vi "Display Lab Panel V6.vi"() -> ()   [LabVIEW 2013]
uses:
  Global display 1.vi
  Global display 2.vi
  Global display 3.vi
panel:
  in  "Tab Control 2":T1(tab)
  out "SIG LAB05-2":T2 {"PF" format="%.2f"; "AMPS" format="%.1f"}
  out "SIG LAB05-1":T2 {"PF" format="%.2f"; "AMPS" format="%.1f"}
  out "SIG LAB04-2":T2 {"PF" format="%.2f"; "AMPS" format="%.1f"}
  out "SIG LAB04-1":T2 {"PF" format="%.2f"; "AMPS" format="%.1f"}
  out "SIG LAB03-2":T2 {"PF" format="%.2f"; "AMPS" format="%.1f"}
  out "SIG LAB03-1":T2 {"PF" format="%.2f"; "AMPS" format="%.1f"}
  out "SIG LAB02-2":T2 {"PF" format="%.2f"; "AMPS" format="%.1f"}
  in  "RUN LAB01-1":bool
  in  "O/I  LAB05-1":bool
  in  "O/I  LAB05-2":bool
  in  "O/I  LAB04-1":bool
  in  "O/I  LAB04-2":bool
  in  "O/I  LAB02-1":bool
  in  "O/I  LAB02-2":bool
  in  "O/I  LAB01-2":bool
  in  "O/I  LAB01-1":bool
  in  "O/I  LAB03-1":bool
  in  "RUN LAB05-2":bool
  in  "RUN LAB05-1":bool
  in  "RUN LAB04-2":bool
  in  "RUN LAB04-1":bool
  in  "RUN LAB03-2":bool
  in  "RUN LAB03-1":bool
  in  "RUN LAB02-2":bool
  in  "RUN LAB02-1":bool
  in  "RUN LAB01-2":bool
  in  "SELECT LAB05-2":T3(radio)
  in  "SELECT LAB05-1":T3(radio)
  in  "SELECT LAB04-2":T3(radio)
  in  "SELECT LAB04-1":T3(radio)
  in  "SELECT LAB03-2":T3(radio)
  in  "SELECT LAB03-1":T3(radio)
  in  "SELECT LAB02-2":T3(radio)
  in  "SELECT LAB02-1":T3(radio)
  in  "SELECT LAB01-2":T3(radio)
  in  "SELECT LAB01-1":T3(radio)
  in  "O/I  LAB03-2":bool
  out "SIG LAB01-1":T2 {"PF" format="%.2f"; "AMPS" format="%.1f"}
  out "SIG LAB01-2":T2 {"PF" format="%.2f"; "AMPS" format="%.1f"}
  out "SIG LAB02-1":T2 {"PF" format="%.2f"; "AMPS" format="%.1f"}
  out "DISP LAB05-2":T4 {"MINS" format="%.2g"}
  out "DISP LAB05-1":T4 {"MINS" format="%.2g"}
  out "DISP LAB04-2":T4 {"MINS" format="%.2g"}
  out "DISP LAB04-1":T4 {"MINS" format="%.2g"}
  out "DISP LAB03-2":T4 {"MINS" format="%.2g"}
  out "DISP LAB03-1":T4 {"MINS" format="%.2g"}
  in  "SET LAB05-2":T5={"NAME"="", "DESCRIPTION"="", "CYCLES"=5.0, "T-RISE mins"=0.0, "T-RISE deg C"=0.0} {"CYCLES" min=5.0 step=1.0}
  in  "SET LAB05-1":T5={"NAME"="", "DESCRIPTION"="", "CYCLES"=5.0, "T-RISE mins"=0.0, "T-RISE deg C"=0.0} {"CYCLES" min=5.0 step=1.0}
  in  "SET LAB04-2":T5={"NAME"="", "DESCRIPTION"="", "CYCLES"=5.0, "T-RISE mins"=0.0, "T-RISE deg C"=0.0} {"CYCLES" min=5.0 step=1.0}
  in  "SET LAB04-1":T5={"NAME"="", "DESCRIPTION"="", "CYCLES"=5.0, "T-RISE mins"=0.0, "T-RISE deg C"=0.0} {"CYCLES" min=5.0 step=1.0}
  in  "SET LAB03-2":T5={"NAME"="", "DESCRIPTION"="", "CYCLES"=5.0, "T-RISE mins"=0.0, "T-RISE deg C"=0.0} {"CYCLES" min=5.0 step=1.0}
  in  "SET LAB03-1":T5={"NAME"="", "DESCRIPTION"="", "CYCLES"=5.0, "T-RISE mins"=0.0, "T-RISE deg C"=0.0} {"CYCLES" min=5.0 step=1.0}
  out "DISP LAB02-2":T4 {"MINS" format="%.2g"}
  out "DISP LAB02-1":T4 {"MINS" format="%.2g"}
  in  "SET LAB02-2":T5={"NAME"="", "DESCRIPTION"="", "CYCLES"=5.0, "T-RISE mins"=0.0, "T-RISE deg C"=0.0} {"CYCLES" min=5.0 step=1.0}
  in  "SET LAB02-1":T5={"NAME"="", "DESCRIPTION"="", "CYCLES"=5.0, "T-RISE mins"=0.0, "T-RISE deg C"=0.0} {"CYCLES" min=5.0 step=1.0}
  out "RESULT LAB05-2":bool
  out "RESULT LAB05-1":bool
  out "RESULT LAB04-2":bool
  out "RESULT LAB04-1":bool
  out "RESULT LAB03-2":bool
  out "RESULT LAB03-1":bool
  out "RESULT LAB02-2":bool
  out "RESULT LAB02-1":bool
  out "RESULT LAB01-2":bool
  out "RESULT LAB01-1":bool
  in  "SET LAB01-1":T5={"NAME"="", "DESCRIPTION"="", "CYCLES"=5.0, "T-RISE mins"=0.0, "T-RISE deg C"=0.0} {"CYCLES" min=5.0 step=1.0}
  in  "SET LAB01-2":T5={"NAME"="", "DESCRIPTION"="", "CYCLES"=5.0, "T-RISE mins"=0.0, "T-RISE deg C"=0.0} {"CYCLES" min=5.0 step=1.0}
  out "DISP LAB01-1":T4 {"MINS" format="%.2g"}
  out "DISP LAB01-2":T4 {"MINS" format="%.2f"}
  in  "Save Log Files\nTo Disk For\nViewing":bool
  out "LOG LAB05-2":string
  out "LOG LAB04-2":string
  out "LOG LAB03-2":string
  out "LOG LAB02-2":string
  out "LOG LAB01-2":string
  out "LOG LAB05-1":string
  out "LOG LAB04-1":string
  out "LOG LAB03-1":string
  out "LOG LAB02-1":string
  out "LOG LAB01-1":string
  out "LAB01 TEMP":dynamicdata(graph)
  out "LAB01 VOLTS":dynamicdata(graph)
  out "LAB01 AMPS":dynamicdata(graph)
  out "LAB02 TEMP":dynamicdata(graph)
  out "LAB02 VOLTS":dynamicdata(graph)
  out "LAB02 AMPS":dynamicdata(graph)
  out "LAB03 TEMP":dynamicdata(graph)
  out "LAB03 VOLTS":dynamicdata(graph)
  out "LAB03 AMPS":dynamicdata(graph)
  out "LAB04 TEMP":dynamicdata(graph)
  out "LAB04 VOLTS":dynamicdata(graph)
  out "LAB04 AMPS":dynamicdata(graph)
  out "LAB05 TEMP":dynamicdata(graph)
  out "LAB05 VOLTS":dynamicdata(graph)
  out "LAB05 AMPS":dynamicdata(graph)
  in  "Stop Button":bool
  out "log file dir":string
  out "log5-2":dbl
  out "log4-2":dbl
  out "log3-2":dbl
  out "log2-2":dbl
  out "log1-2":dbl
  out "log5-1":dbl
  out "log4-1":dbl
  out "log3-1":dbl
  out "log2-1":dbl
  out "log1-1":dbl
  out "graph update":bool
  out "LF5-2":bool
  out "LF5-1":bool
  out "LF3-2":bool
  out "LF3-1":bool
  out "LF4-2":bool
  out "LF4-1":bool
  out "LF2-2":bool
  out "LF2-1":bool
  out "LF1-2":bool
  out "LF1-1":bool
  out "error out":errorcluster
  # "LAB01"
  # "LAB02"
  # "LAB05"
  # "LAB03"
  # "LAB04"
  # "LAB01"
  # "LAB02"
  # "LAB03"
  # "LAB04"
  # "LAB05"
  # "PANEL ID / DATE / TIME / DESCRIPTION / CYCLES / TEST TIME / STATUS"
  # "PANEL ID / DATE / TIME / DESCRIPTION / CYCLES / TEST TIME / STATUS"
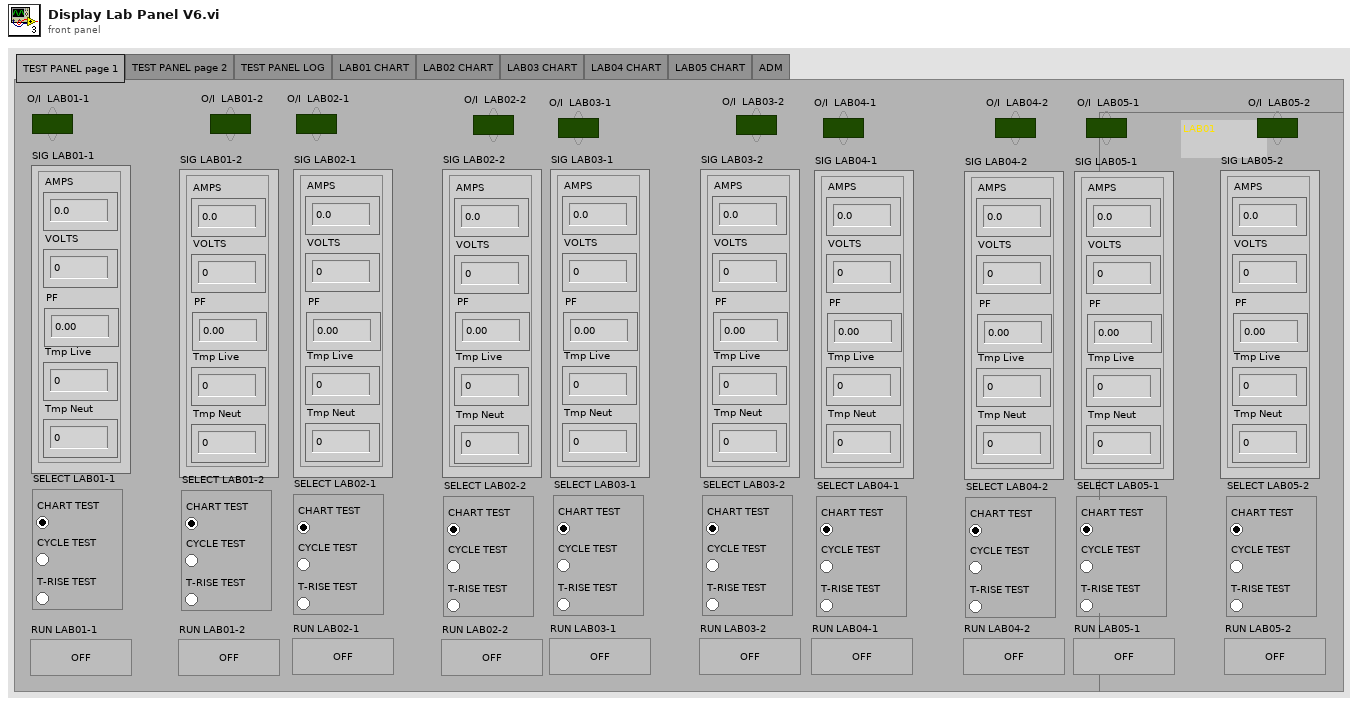
[diagram p1: front panel]
types:
  T1 = enum32{"TEST PANEL page 1", "TEST PANEL page 2", "TEST PANEL LOG", "LAB01 CHART", "LAB02 CHART", "LAB03 CHART", "LAB04 CHART", "LAB05 CHART", "ADM"}
  T2 = cluster{"AMPS":dbl, "VOLTS":dbl, "PF":dbl, "Tmp Live":dbl, "Tmp Neut":dbl}
  T3 = enum32{"CHART TEST", "CYCLE TEST", "T-RISE TEST"}
  T4 = cluster{"CYCLE":dbl, "MINS":dbl, "STATUS":string}
  T5 = cluster{"NAME":string, "DESCRIPTION":string, "CYCLES":dbl, "T-RISE mins":dbl, "T-RISE deg C":dbl}
  T6 = enum8{"Enabled", "Disabled", "Disabled and Grayed Out"}
  T7 = cluster{string, "date string":string, "time string":string, "DESCRIPTION":string, string, string, "STATUS":string}
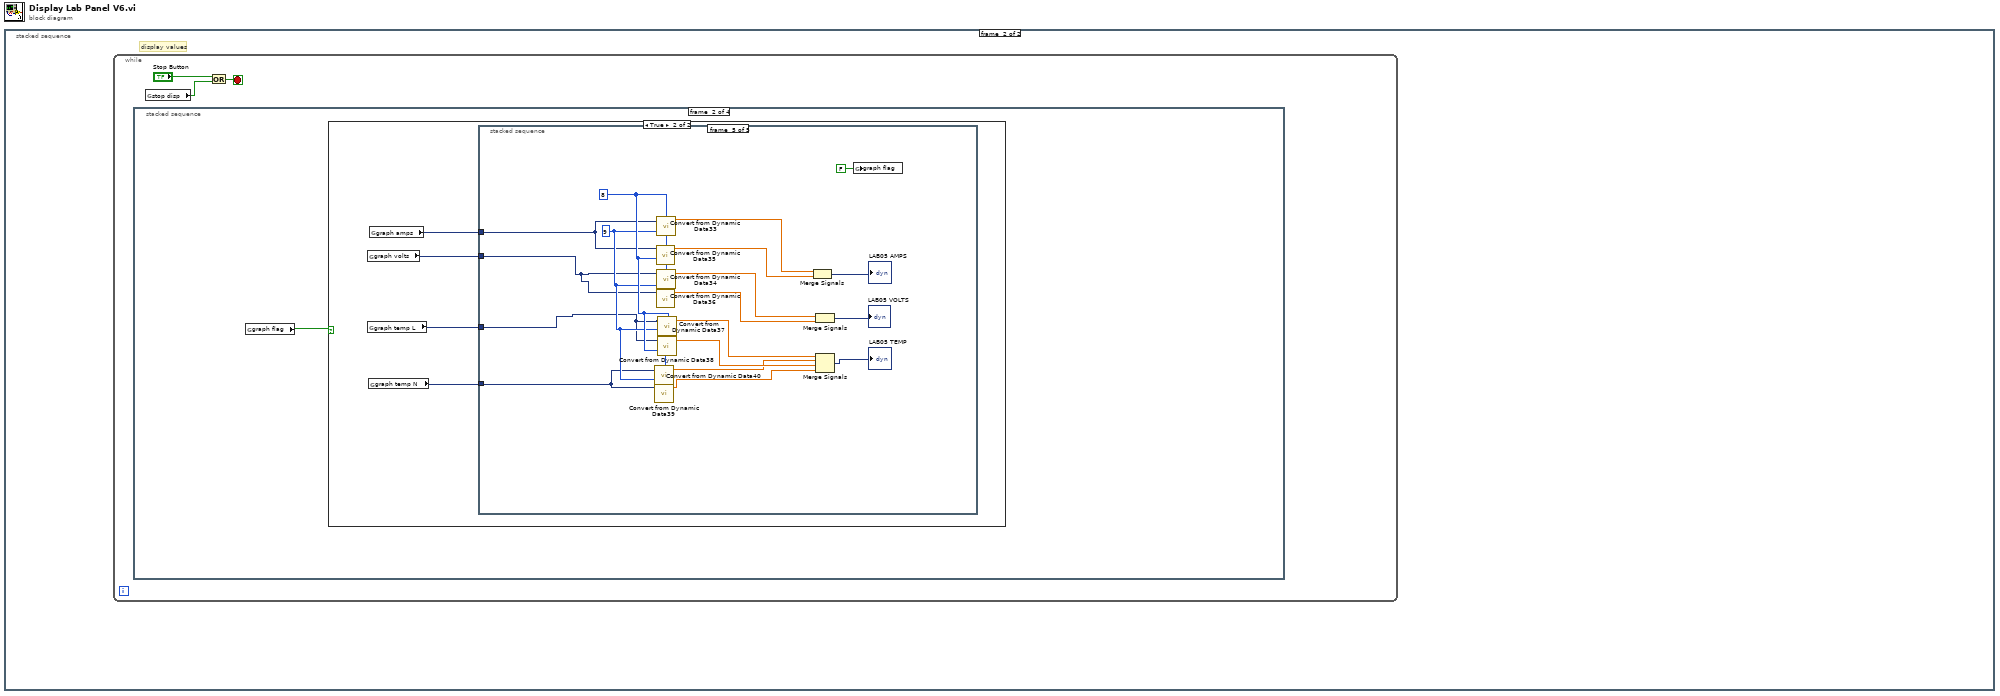
[diagram p0: block diagram]
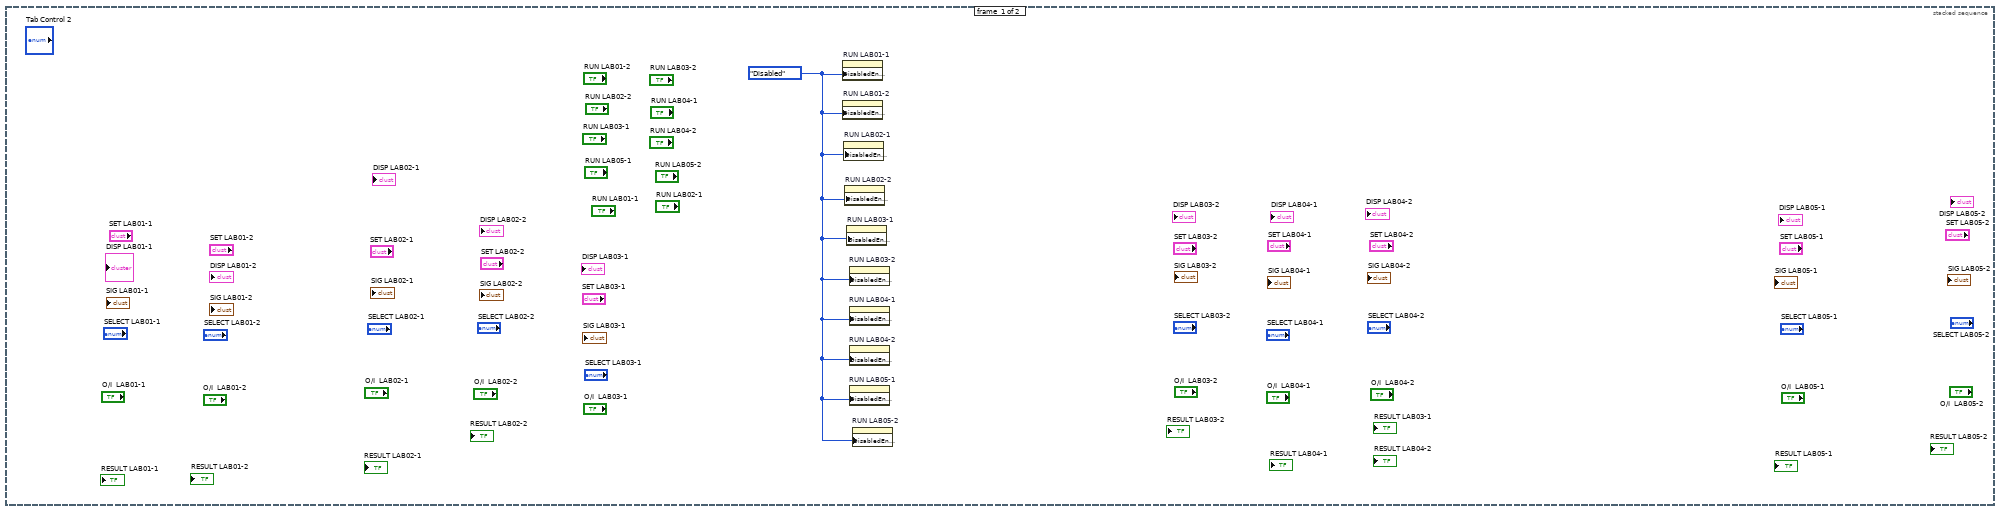
[diagram p2: hidden frame]
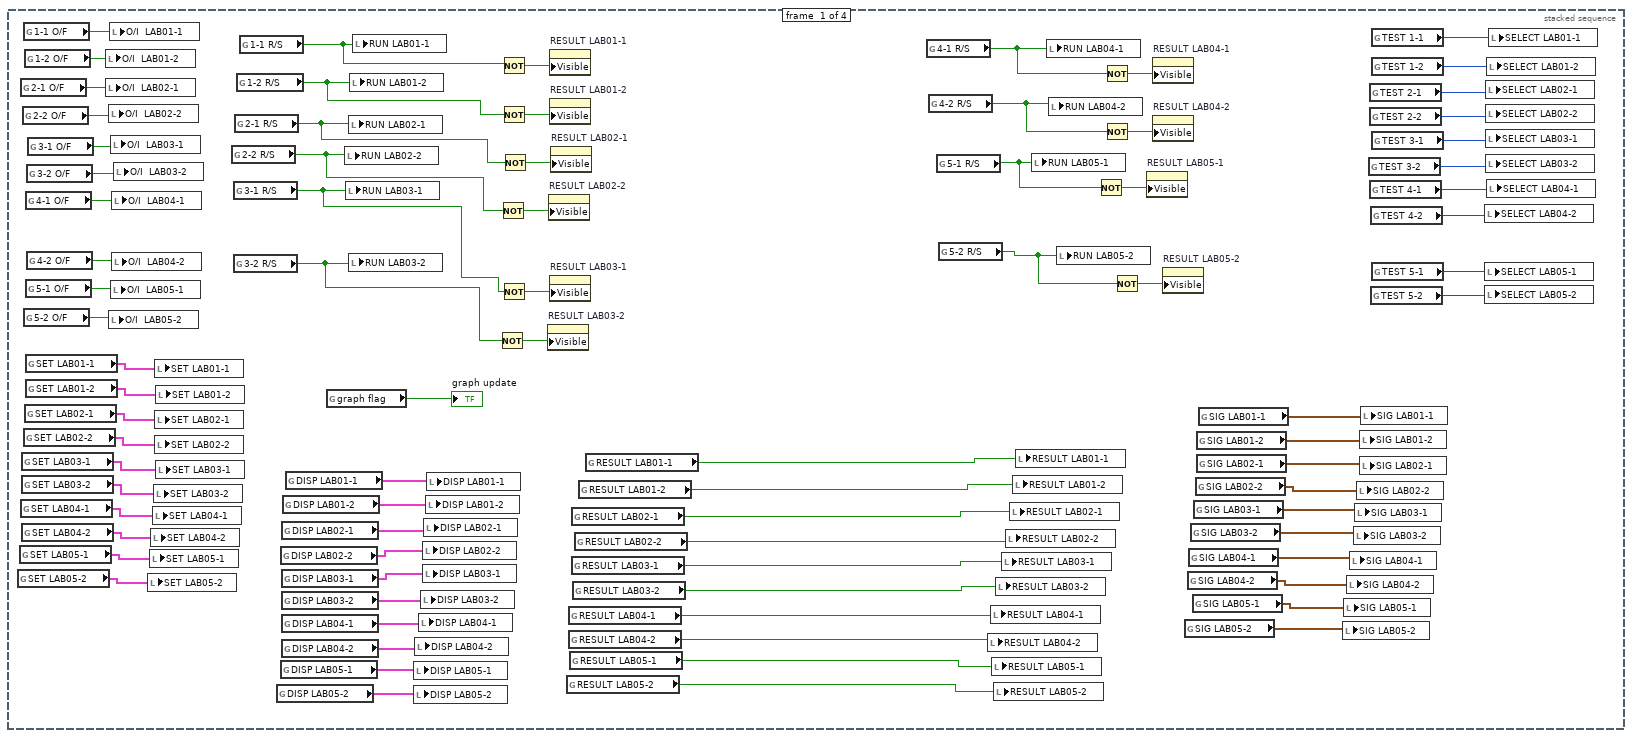
[diagram p3: hidden frame]
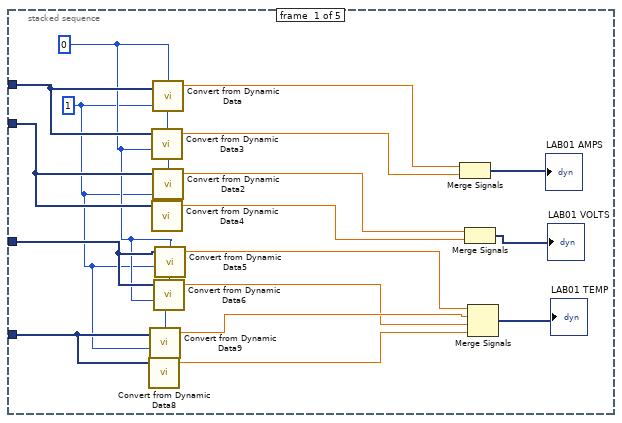
[diagram p5: hidden frame]
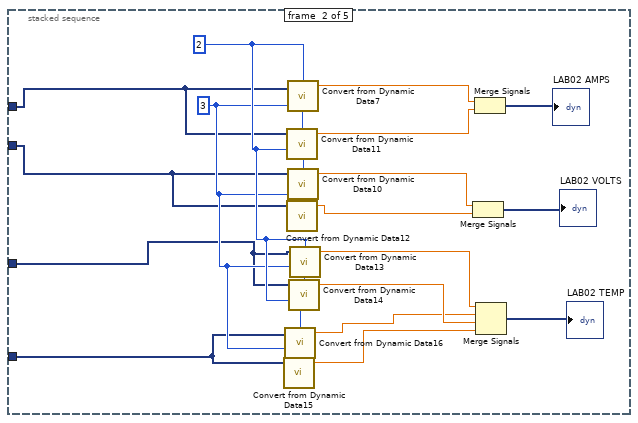
[diagram p6: hidden frame]
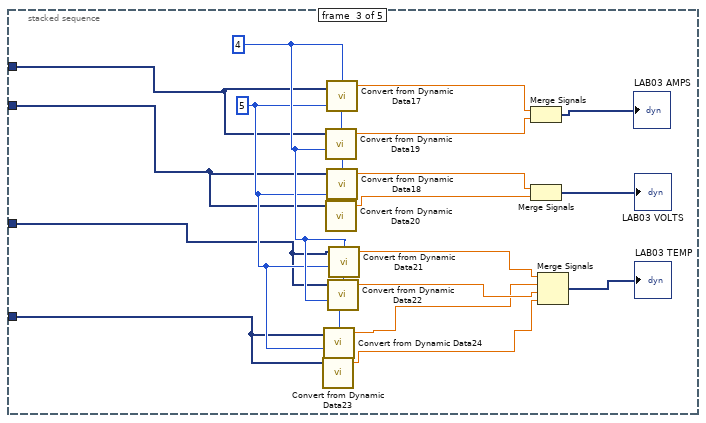
[diagram p7: hidden frame]
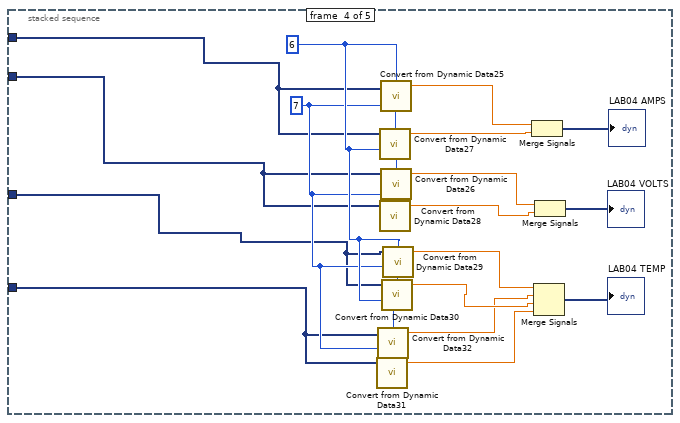
[diagram p8: hidden frame]
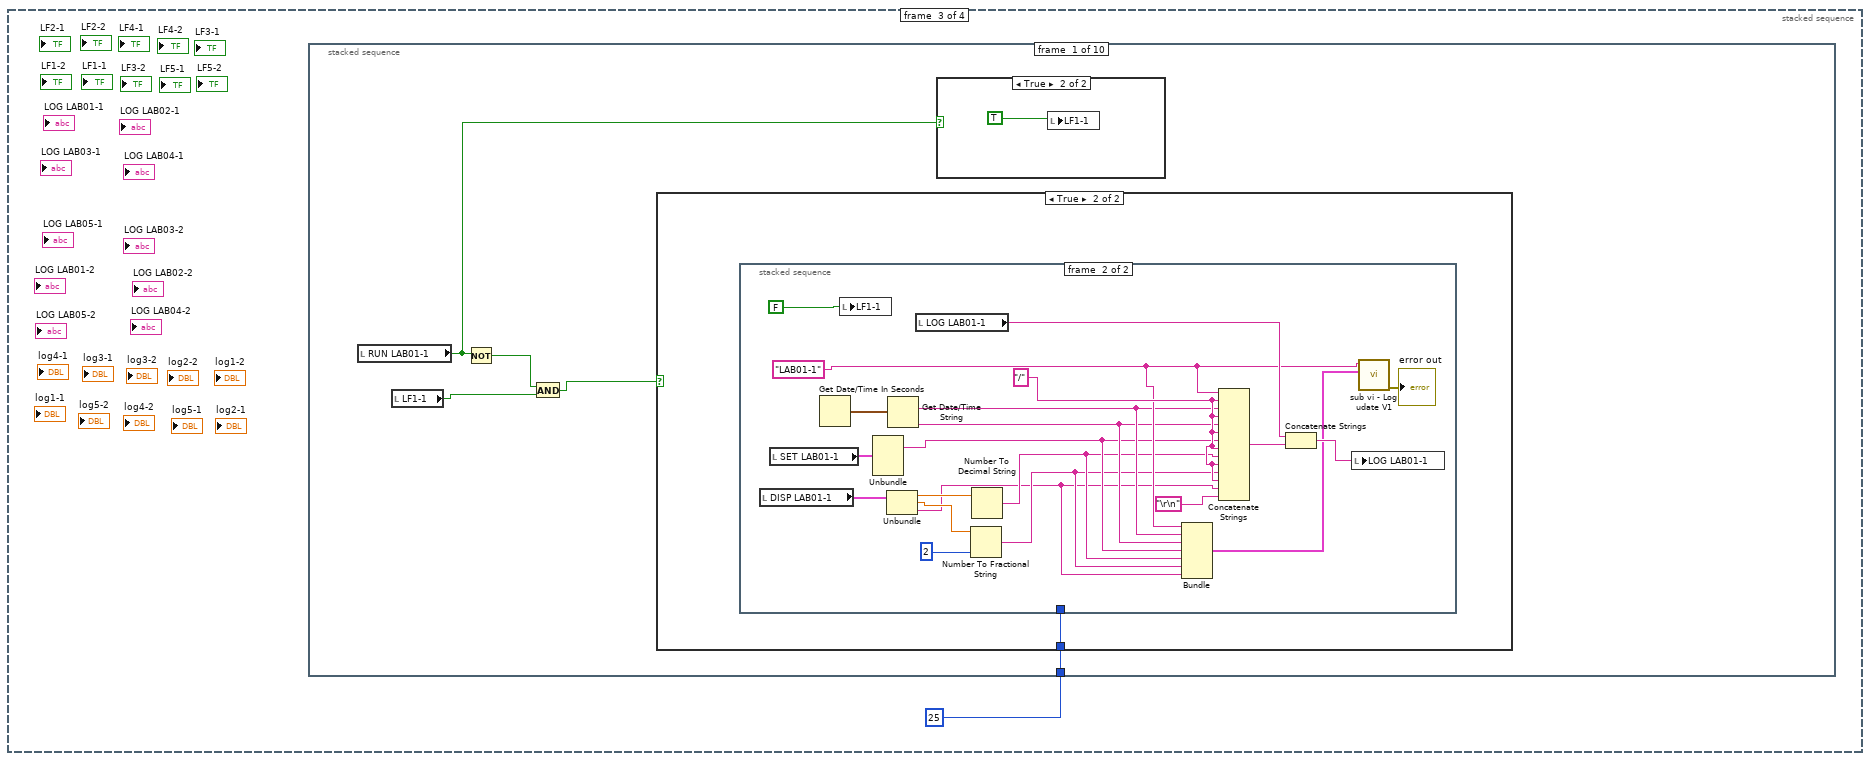
[diagram p9: hidden frame]
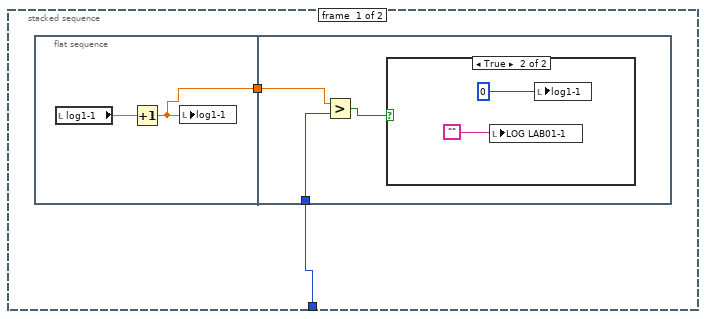
[diagram p11: hidden frame]
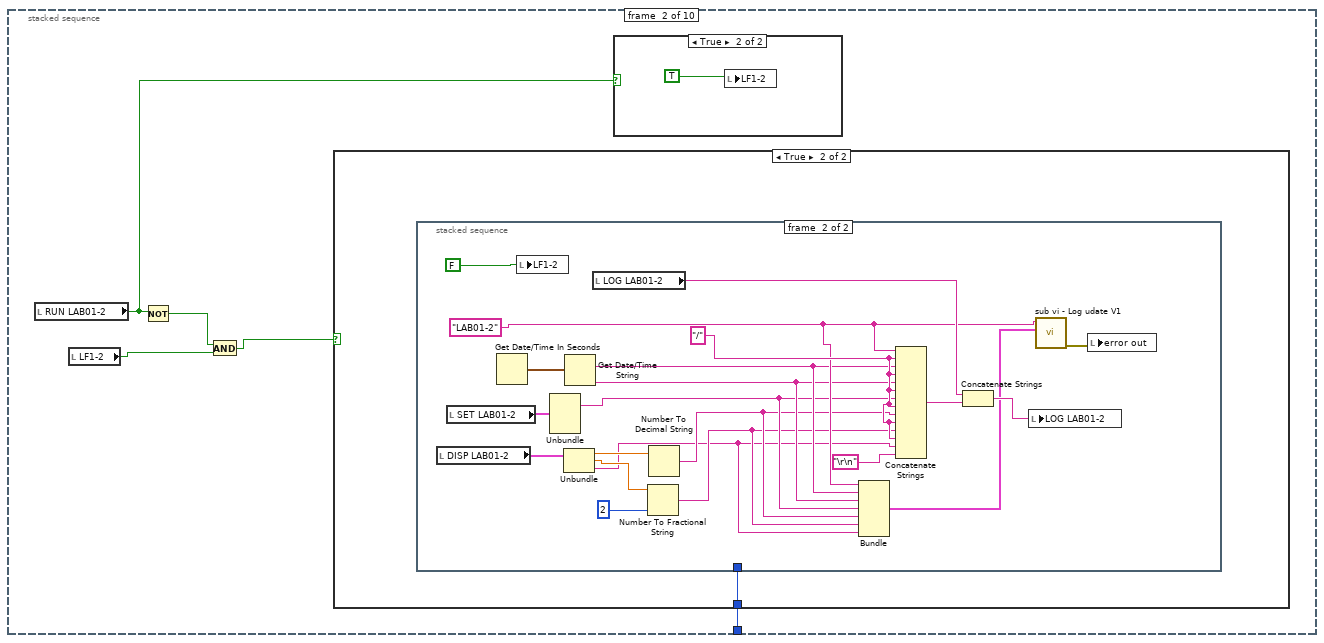
[diagram p14: hidden frame]
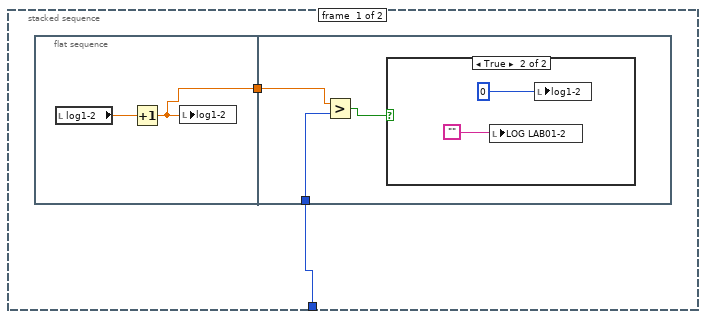
[diagram p16: hidden frame]
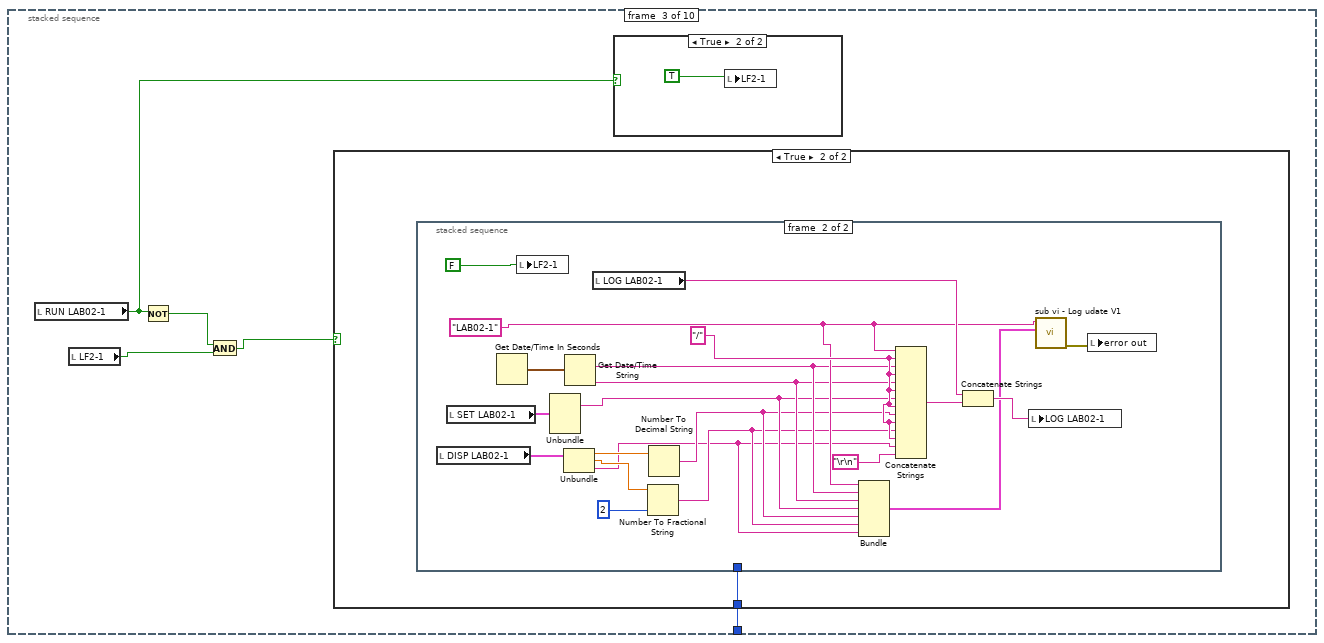
[diagram p19: hidden frame]
diagram:
  n1 = stacked-sequence {
    frame #0 {
      w1 = T6."Disabled" ("Disabled")
      n2 = property on="RUN LAB01-1" class="Bool (strict)"("DisabledEnum"=w1) -> ()  [unwired: 2 in, 2 out]
      n3 = property on="RUN LAB01-2" class="Bool (strict)"("DisabledEnum"=w1) -> ()  [unwired: 2 in, 2 out]
      n4 = property on="RUN LAB02-1" class="Bool (strict)"("DisabledEnum"=w1) -> ()  [unwired: 2 in, 2 out]
      n5 = property on="RUN LAB02-2" class="Bool (strict)"("DisabledEnum"=w1) -> ()  [unwired: 2 in, 2 out]
      n6 = property on="RUN LAB03-1" class="Bool (strict)"("DisabledEnum"=w1) -> ()  [unwired: 2 in, 2 out]
      n7 = property on="RUN LAB03-2" class="Bool (strict)"("DisabledEnum"=w1) -> ()  [unwired: 2 in, 2 out]
      n8 = property on="RUN LAB04-1" class="Bool (strict)"("DisabledEnum"=w1) -> ()  [unwired: 2 in, 2 out]
      n9 = property on="RUN LAB04-2" class="Bool (strict)"("DisabledEnum"=w1) -> ()  [unwired: 2 in, 2 out]
      n10 = property on="RUN LAB05-1" class="Bool (strict)"("DisabledEnum"=w1) -> ()  [unwired: 2 in, 2 out]
      n11 = property on="RUN LAB05-2" class="Bool (strict)"("DisabledEnum"=w1) -> ()  [unwired: 2 in, 2 out]
    }
    frame #1 {
      # "display values"
      n12 = while {
        stop <- w4 stop-if-true
        n13 = stacked-sequence {
          frame #0 {
            n14 = global read "Global display 2.vi" "SET LAB05-2"() -> (w46:T5)
            n15 = global read "Global display 2.vi" "SET LAB05-1"() -> (w47:T5)
            n16 = global read "Global display 1.vi" "2-1 O/F"() -> (w83:bool)
            n17 = global read "Global display 2.vi" "SET LAB04-1"() -> (w49:T5)
            n18 = global read "Global display 2.vi" "SET LAB03-1"() -> (w51:T5)
            n19 = global read "Global display 2.vi" "SET LAB03-2"() -> (w50:T5)
            n20 = global read "Global display 2.vi" "SET LAB04-2"() -> (w48:T5)
            n21 = global read "Global display 1.vi" "2-2 O/F"() -> (w82:bool)
            n22 = global read "Global display 1.vi" "1-1 O/F"() -> (w85:bool)
            n23 = global read "Global display 1.vi" "5-2 O/F"() -> (w76:bool)
            n24 = global read "Global display 2.vi" "SET LAB02-2"() -> (w52:T5)
            n25 = global read "Global display 1.vi" "1-2 O/F"() -> (w84:bool)
            n26 = global read "Global display 2.vi" "SET LAB02-1"() -> (w53:T5)
            n27 = global read "Global display 1.vi" "4-1 O/F"() -> (w79:bool)
            n28 = global read "Global display 1.vi" "5-1 O/F"() -> (w77:bool)
            n29 = global read "Global display 2.vi" "SET LAB01-1"() -> (w55:T5)
            n30 = global read "Global display 2.vi" "SET LAB01-2"() -> (w54:T5)
            n31 = global read "Global display 1.vi" "3-2 O/F"() -> (w80:bool)
            n32 = global read "Global display 1.vi" "4-2 O/F"() -> (w78:bool)
            n33 = global read "Global display 1.vi" "3-1 O/F"() -> (w81:bool)
            n34 = local write "O/I  LAB01-2"(w84) -> ()
            n35 = local write "O/I  LAB02-1"(w83) -> ()
            n36 = local write "O/I  LAB02-2"(w82) -> ()
            n37 = local write "O/I  LAB05-2"(w76) -> ()
            n38 = local write "O/I  LAB01-1"(w85) -> ()
            n39 = local write "O/I  LAB03-1"(w81) -> ()
            n40 = local write "O/I  LAB05-1"(w77) -> ()
            n41 = local write "O/I  LAB04-1"(w79) -> ()
            n42 = local write "O/I  LAB04-2"(w78) -> ()
            n43 = local write "O/I  LAB03-2"(w80) -> ()
            n44 = local write "SET LAB05-2"(w46) -> ()
            n45 = local write "SET LAB05-1"(w47) -> ()
            n46 = local write "SET LAB04-2"(w48) -> ()
            n47 = local write "SET LAB04-1"(w49) -> ()
            n48 = local write "SET LAB03-2"(w50) -> ()
            n49 = local write "SET LAB01-1"(w55) -> ()
            n50 = local write "SET LAB02-1"(w53) -> ()
            n51 = local write "SET LAB02-2"(w52) -> ()
            n52 = local write "SET LAB01-2"(w54) -> ()
            n53 = local write "SET LAB03-1"(w51) -> ()
            n54 = global read "Global display 1.vi" "2-2 R/S"() -> (w16:bool)
            n55 = global read "Global display 1.vi" "3-1 R/S"() -> (w15:bool)
            n56 = global read "Global display 1.vi" "3-2 R/S"() -> (w14:bool)
            n57 = global read "Global display 1.vi" "2-1 R/S"() -> (w17:bool)
            n58 = global read "Global display 1.vi" "1-2 R/S"() -> (w18:bool)
            n59 = global read "Global display 1.vi" "1-1 R/S"() -> (w24:bool)
            n60 = global read "Global display 2.vi" "DISP LAB05-2"() -> (w36:T4)
            n61 = global read "Global display 2.vi" "DISP LAB02-2"() -> (w42:T4)
            n62 = global read "Global display 2.vi" "DISP LAB05-1"() -> (w37:T4)
            n63 = global read "Global display 2.vi" "DISP LAB02-1"() -> (w43:T4)
            n64 = global read "Global display 2.vi" "DISP LAB03-1"() -> (w41:T4)
            n65 = global read "Global display 2.vi" "DISP LAB03-2"() -> (w40:T4)
            n66 = global read "Global display 2.vi" "DISP LAB04-1"() -> (w39:T4)
            n67 = global read "Global display 2.vi" "DISP LAB04-2"() -> (w38:T4)
            n68 = global read "Global display 2.vi" "DISP LAB01-2"() -> (w44:T4)
            n69 = global read "Global display 2.vi" "DISP LAB01-1"() -> (w45:T4)
            n70 = global read "Global display 3.vi" "graph flag"() -> (→"graph update":bool)
            n71 = local write "RUN LAB02-2"(w16) -> ()
            n72 = local write "RUN LAB03-1"(w15) -> ()
            n73 = local write "RUN LAB02-1"(w17) -> ()
            n74 = local write "RUN LAB03-2"(w14) -> ()
            n75 = local write "RUN LAB01-2"(w18) -> ()
            n76 = local write "RUN LAB01-1"(w24) -> ()
            n77 = local write "DISP LAB05-1"(w37) -> ()
            n78 = local write "DISP LAB05-2"(w36) -> ()
            n79 = local write "DISP LAB04-2"(w38) -> ()
            n80 = local write "DISP LAB04-1"(w39) -> ()
            n81 = local write "DISP LAB03-2"(w40) -> ()
            n82 = local write "DISP LAB02-2"(w42) -> ()
            n83 = local write "DISP LAB03-1"(w41) -> ()
            n84 = local write "DISP LAB02-1"(w43) -> ()
            n85 = local write "DISP LAB01-2"(w44) -> ()
            n86 = local write "DISP LAB01-1"(w45) -> ()
            n87 = Not(x=w14) -> (.not. x?=w19:bool)
            n88 = Not(x=w16) -> (.not. x?=w21:bool)
            n89 = Not(x=w24) -> (.not. x?=w25:bool)
            n90 = Not(x=w18) -> (.not. x?=w23:bool)
            n91 = Not(x=w15) -> (.not. x?=w20:bool)
            n92 = Not(x=w17) -> (.not. x?=w22:bool)
            n93 = property on="RESULT LAB03-2" class="Bool (strict)"("Visible"=w19) -> ()  [unwired: 2 in, 2 out]
            n94 = property on="RESULT LAB02-2" class="Bool (strict)"("Visible"=w21) -> ()  [unwired: 2 in, 2 out]
            n95 = property on="RESULT LAB01-1" class="Bool (strict)"("Visible"=w25) -> ()  [unwired: 2 in, 2 out]
            n96 = property on="RESULT LAB01-2" class="Bool (strict)"("Visible"=w23) -> ()  [unwired: 2 in, 2 out]
            n97 = property on="RESULT LAB03-1" class="Bool (strict)"("Visible"=w20) -> ()  [unwired: 2 in, 2 out]
            n98 = property on="RESULT LAB02-1" class="Bool (strict)"("Visible"=w22) -> ()  [unwired: 2 in, 2 out]
            n99 = global read "Global display 2.vi" "RESULT LAB05-2"() -> (w26:bool)
            n100 = global read "Global display 2.vi" "RESULT LAB04-1"() -> (w29:bool)
            n101 = global read "Global display 2.vi" "RESULT LAB04-2"() -> (w28:bool)
            n102 = global read "Global display 2.vi" "RESULT LAB05-1"() -> (w27:bool)
            n103 = global read "Global display 2.vi" "RESULT LAB02-1"() -> (w33:bool)
            n104 = global read "Global display 2.vi" "RESULT LAB03-1"() -> (w31:bool)
            n105 = global read "Global display 2.vi" "RESULT LAB03-2"() -> (w30:bool)
            n106 = global read "Global display 2.vi" "RESULT LAB02-2"() -> (w32:bool)
            n107 = global read "Global display 2.vi" "RESULT LAB01-2"() -> (w34:bool)
            n108 = global read "Global display 2.vi" "RESULT LAB01-1"() -> (w35:bool)
            n109 = global read "Global display 1.vi" "4-1 R/S"() -> (w12:bool)
            n110 = global read "Global display 1.vi" "4-2 R/S"() -> (w10:bool)
            n111 = global read "Global display 1.vi" "5-1 R/S"() -> (w8:bool)
            n112 = global read "Global display 1.vi" "5-2 R/S"() -> (w6:bool)
            n113 = local write "RESULT LAB04-2"(w28) -> ()
            n114 = local write "RESULT LAB04-1"(w29) -> ()
            n115 = local write "RESULT LAB05-1"(w27) -> ()
            n116 = local write "RESULT LAB05-2"(w26) -> ()
            n117 = local write "RESULT LAB03-2"(w30) -> ()
            n118 = local write "RESULT LAB03-1"(w31) -> ()
            n119 = local write "RESULT LAB02-2"(w32) -> ()
            n120 = local write "RESULT LAB02-1"(w33) -> ()
            n121 = local write "RESULT LAB01-2"(w34) -> ()
            n122 = local write "RESULT LAB01-1"(w35) -> ()
            n123 = local write "RUN LAB05-1"(w8) -> ()
            n124 = local write "RUN LAB04-1"(w12) -> ()
            n125 = local write "RUN LAB04-2"(w10) -> ()
            n126 = local write "RUN LAB05-2"(w6) -> ()
            n127 = Not(x=w8) -> (.not. x?=w9:bool)
            n128 = Not(x=w12) -> (.not. x?=w13:bool)
            n129 = Not(x=w10) -> (.not. x?=w11:bool)
            n130 = Not(x=w6) -> (.not. x?=w7:bool)
            n131 = property on="RESULT LAB05-1" class="Bool (strict)"("Visible"=w9) -> ()  [unwired: 2 in, 2 out]
            n132 = property on="RESULT LAB04-1" class="Bool (strict)"("Visible"=w13) -> ()  [unwired: 2 in, 2 out]
            n133 = property on="RESULT LAB04-2" class="Bool (strict)"("Visible"=w11) -> ()  [unwired: 2 in, 2 out]
            n134 = property on="RESULT LAB05-2" class="Bool (strict)"("Visible"=w7) -> ()  [unwired: 2 in, 2 out]
            n135 = global read "Global display 1.vi" "SIG LAB05-2"() -> (w56:T2)
            n136 = global read "Global display 1.vi" "SIG LAB04-2"() -> (w58:T2)
            n137 = global read "Global display 1.vi" "SIG LAB04-1"() -> (w59:T2)
            n138 = global read "Global display 1.vi" "SIG LAB03-2"() -> (w60:T2)
            n139 = global read "Global display 1.vi" "SIG LAB05-1"() -> (w57:T2)
            n140 = global read "Global display 1.vi" "SIG LAB03-1"() -> (w61:T2)
            n141 = global read "Global display 1.vi" "SIG LAB02-2"() -> (w62:T2)
            n142 = global read "Global display 1.vi" "SIG LAB01-2"() -> (w64:T2)
            n143 = global read "Global display 1.vi" "SIG LAB02-1"() -> (w63:T2)
            n144 = global read "Global display 1.vi" "SIG LAB01-1"() -> (w65:T2)
            n145 = local write "SIG LAB05-2"(w56) -> ()
            n146 = local write "SIG LAB05-1"(w57) -> ()
            n147 = local write "SIG LAB04-2"(w58) -> ()
            n148 = local write "SIG LAB04-1"(w59) -> ()
            n149 = local write "SIG LAB03-2"(w60) -> ()
            n150 = local write "SIG LAB03-1"(w61) -> ()
            n151 = local write "SIG LAB02-2"(w62) -> ()
            n152 = local write "SIG LAB01-2"(w64) -> ()
            n153 = local write "SIG LAB02-1"(w63) -> ()
            n154 = local write "SIG LAB01-1"(w65) -> ()
            n155 = global read "Global display 1.vi" "TEST 3-2"() -> (w70:T3)
            n156 = global read "Global display 1.vi" "TEST 2-1"() -> (w73:T3)
            n157 = global read "Global display 1.vi" "TEST 2-2"() -> (w72:T3)
            n158 = global read "Global display 1.vi" "TEST 4-1"() -> (w69:T3)
            n159 = global read "Global display 1.vi" "TEST 4-2"() -> (w68:T3)
            n160 = global read "Global display 1.vi" "TEST 5-2"() -> (w66:T3)
            n161 = global read "Global display 1.vi" "TEST 1-1"() -> (w75:T3)
            n162 = global read "Global display 1.vi" "TEST 1-2"() -> (w74:T3)
            n163 = global read "Global display 1.vi" "TEST 3-1"() -> (w71:T3)
            n164 = global read "Global display 1.vi" "TEST 5-1"() -> (w67:T3)
            n165 = local write "SELECT LAB04-2"(w68) -> ()
            n166 = local write "SELECT LAB05-1"(w67) -> ()
            n167 = local write "SELECT LAB05-2"(w66) -> ()
            n168 = local write "SELECT LAB02-1"(w73) -> ()
            n169 = local write "SELECT LAB02-2"(w72) -> ()
            n170 = local write "SELECT LAB03-1"(w71) -> ()
            n171 = local write "SELECT LAB03-2"(w70) -> ()
            n172 = local write "SELECT LAB01-2"(w74) -> ()
            n173 = local write "SELECT LAB04-1"(w69) -> ()
            n174 = local write "SELECT LAB01-1"(w75) -> ()
          }
          frame #1 {
            n175 = global read "Global display 3.vi" "graph flag"() -> (w86:bool)
            n176 = case shown="True" w86 {
              frame False {
              }
              frame True {
                n177 = global read "Global display 3.vi" "graph volts"() -> (w89:dynamicdata)
                n178 = global read "Global display 3.vi" "graph temp L"() -> (w88:dynamicdata)
                n179 = global read "Global display 3.vi" "graph temp N"() -> (w87:dynamicdata)
                n180 = global read "Global display 3.vi" "graph amps"() -> (w90:dynamicdata)
                n181 = stacked-sequence {
                  tunnel: w90 -> [w104 w119 w136 w153 w170]
                  tunnel: w89 -> [w101 w116 w135 w152 w169]
                  tunnel: w88 -> [w98 w118 w134 w151 w168]
                  tunnel: w87 -> [w97 w117 w133 w150 w167]
                  frame #0 {
                    w91 = 1
                    w96 = 0
                    n182 = call "Convert from Dynamic Data8"("Dynamic Data Type"=w97, "Channel"=w91) -> ("Scalar"=w92:dbl)  [unwired: 2 in]
                    n183 = call "Convert from Dynamic Data9"("Dynamic Data Type"=w97, "Channel"=w96) -> ("Scalar"=w94:dbl)  [unwired: 2 in]
                    n184 = call "Convert from Dynamic Data3"("Dynamic Data Type"=w104, "Channel"=w91) -> ("Scalar"=w102:dbl)  [unwired: 2 in]
                    n185 = call "Convert from Dynamic Data4"("Dynamic Data Type"=w101, "Channel"=w91) -> ("Scalar"=w99:dbl)  [unwired: 2 in]
                    n186 = call "Convert from Dynamic Data"("Dynamic Data Type"=w104, "Channel"=w96) -> ("Scalar"=w103:dbl)  [unwired: 2 in]
                    n187 = call "Convert from Dynamic Data2"("Dynamic Data Type"=w101, "Channel"=w96) -> ("Scalar"=w100:dbl)  [unwired: 2 in]
                    n188 = call "Convert from Dynamic Data6"("Dynamic Data Type"=w98, "Channel"=w91) -> ("Scalar"=w93:dbl)  [unwired: 2 in]
                    n189 = call "Convert from Dynamic Data5"("Dynamic Data Type"=w98, "Channel"=w96) -> ("Scalar"=w95:dbl)  [unwired: 2 in]
                    n190 = Merge Signals(w103, w102) -> (→"LAB01 AMPS":dynamicdata)
                    n191 = Merge Signals(w100, w99) -> (→"LAB01 VOLTS":dynamicdata)
                    n192 = Merge Signals(w95, w94, w93, w92) -> (→"LAB01 TEMP":dynamicdata)
                  }
                  frame #1 {
                    w123 = 3
                    w124 = 2
                    n193 = call "Convert from Dynamic Data15"("Dynamic Data Type"=w117, "Channel"=w123) -> ("Scalar"=w108:dbl)  [unwired: 2 in]
                    n194 = call "Convert from Dynamic Data16"("Dynamic Data Type"=w117, "Channel"=w124) -> ("Scalar"=w109:dbl)  [unwired: 2 in]
                    n195 = call "Convert from Dynamic Data11"("Dynamic Data Type"=w119, "Channel"=w123) -> ("Scalar"=w114:dbl)  [unwired: 2 in]
                    n196 = call "Convert from Dynamic Data12"("Dynamic Data Type"=w116, "Channel"=w123) -> ("Scalar"=w112:dbl)  [unwired: 2 in]
                    n197 = call "Convert from Dynamic Data7"("Dynamic Data Type"=w119, "Channel"=w124) -> ("Scalar"=w115:dbl)  [unwired: 2 in]
                    n198 = call "Convert from Dynamic Data10"("Dynamic Data Type"=w116, "Channel"=w124) -> ("Scalar"=w113:dbl)  [unwired: 2 in]
                    n199 = call "Convert from Dynamic Data14"("Dynamic Data Type"=w118, "Channel"=w123) -> ("Scalar"=w110:dbl)  [unwired: 2 in]
                    n200 = call "Convert from Dynamic Data13"("Dynamic Data Type"=w118, "Channel"=w124) -> ("Scalar"=w111:dbl)  [unwired: 2 in]
                    n201 = Merge Signals(w113, w112) -> (→"LAB02 VOLTS":dynamicdata)
                    n202 = Merge Signals(w115, w114) -> (→"LAB02 AMPS":dynamicdata)
                    n203 = Merge Signals(w111, w109, w110, w108) -> (→"LAB02 TEMP":dynamicdata)
                  }
                  frame #2 {
                    w140 = 5
                    w141 = 4
                    n204 = call "Convert from Dynamic Data23"("Dynamic Data Type"=w133, "Channel"=w140) -> ("Scalar"=w125:dbl)  [unwired: 2 in]
                    n205 = call "Convert from Dynamic Data24"("Dynamic Data Type"=w133, "Channel"=w141) -> ("Scalar"=w126:dbl)  [unwired: 2 in]
                    n206 = call "Convert from Dynamic Data19"("Dynamic Data Type"=w136, "Channel"=w140) -> ("Scalar"=w131:dbl)  [unwired: 2 in]
                    n207 = call "Convert from Dynamic Data20"("Dynamic Data Type"=w135, "Channel"=w140) -> ("Scalar"=w129:dbl)  [unwired: 2 in]
                    n208 = call "Convert from Dynamic Data17"("Dynamic Data Type"=w136, "Channel"=w141) -> ("Scalar"=w132:dbl)  [unwired: 2 in]
                    n209 = call "Convert from Dynamic Data18"("Dynamic Data Type"=w135, "Channel"=w141) -> ("Scalar"=w130:dbl)  [unwired: 2 in]
                    n210 = call "Convert from Dynamic Data22"("Dynamic Data Type"=w134, "Channel"=w140) -> ("Scalar"=w127:dbl)  [unwired: 2 in]
                    n211 = call "Convert from Dynamic Data21"("Dynamic Data Type"=w134, "Channel"=w141) -> ("Scalar"=w128:dbl)  [unwired: 2 in]
                    n212 = Merge Signals(w132, w131) -> (→"LAB03 AMPS":dynamicdata)
                    n213 = Merge Signals(w130, w129) -> (→"LAB03 VOLTS":dynamicdata)
                    n214 = Merge Signals(w128, w126, w127, w125) -> (→"LAB03 TEMP":dynamicdata)
                  }
                  frame #3 {
                    w154 = 7
                    w155 = 6
                    n215 = call "Convert from Dynamic Data31"("Dynamic Data Type"=w150, "Channel"=w154) -> ("Scalar"=w142:dbl)  [unwired: 2 in]
                    n216 = call "Convert from Dynamic Data32"("Dynamic Data Type"=w150, "Channel"=w155) -> ("Scalar"=w143:dbl)  [unwired: 2 in]
                    n217 = call "Convert from Dynamic Data27"("Dynamic Data Type"=w153, "Channel"=w154) -> ("Scalar"=w148:dbl)  [unwired: 2 in]
                    n218 = call "Convert from Dynamic Data28"("Dynamic Data Type"=w152, "Channel"=w154) -> ("Scalar"=w146:dbl)  [unwired: 2 in]
                    n219 = call "Convert from Dynamic Data25"("Dynamic Data Type"=w153, "Channel"=w155) -> ("Scalar"=w149:dbl)  [unwired: 2 in]
                    n220 = call "Convert from Dynamic Data26"("Dynamic Data Type"=w152, "Channel"=w155) -> ("Scalar"=w147:dbl)  [unwired: 2 in]
                    n221 = call "Convert from Dynamic Data30"("Dynamic Data Type"=w151, "Channel"=w154) -> ("Scalar"=w144:dbl)  [unwired: 2 in]
                    n222 = call "Convert from Dynamic Data29"("Dynamic Data Type"=w151, "Channel"=w155) -> ("Scalar"=w145:dbl)  [unwired: 2 in]
                    n223 = Merge Signals(w149, w148) -> (→"LAB04 AMPS":dynamicdata)
                    n224 = Merge Signals(w145, w143, w144, w142) -> (→"LAB04 TEMP":dynamicdata)
                    n225 = Merge Signals(w147, w146) -> (→"LAB04 VOLTS":dynamicdata)
                  }
                  frame #4 {
                    w174 = 9
                    w175 = 8
                    n226 = call "Convert from Dynamic Data39"("Dynamic Data Type"=w167, "Channel"=w174) -> ("Scalar"=w159:dbl)  [unwired: 2 in]
                    n227 = call "Convert from Dynamic Data40"("Dynamic Data Type"=w167, "Channel"=w175) -> ("Scalar"=w160:dbl)  [unwired: 2 in]
                    n228 = call "Convert from Dynamic Data35"("Dynamic Data Type"=w170, "Channel"=w174) -> ("Scalar"=w165:dbl)  [unwired: 2 in]
                    n229 = call "Convert from Dynamic Data36"("Dynamic Data Type"=w169, "Channel"=w174) -> ("Scalar"=w163:dbl)  [unwired: 2 in]
                    n230 = call "Convert from Dynamic Data33"("Dynamic Data Type"=w170, "Channel"=w175) -> ("Scalar"=w166:dbl)  [unwired: 2 in]
                    n231 = call "Convert from Dynamic Data34"("Dynamic Data Type"=w169, "Channel"=w175) -> ("Scalar"=w164:dbl)  [unwired: 2 in]
                    n232 = call "Convert from Dynamic Data38"("Dynamic Data Type"=w168, "Channel"=w174) -> ("Scalar"=w161:dbl)  [unwired: 2 in]
                    n233 = call "Convert from Dynamic Data37"("Dynamic Data Type"=w168, "Channel"=w175) -> ("Scalar"=w162:dbl)  [unwired: 2 in]
                    n234 = Merge Signals(w166, w165) -> (→"LAB05 AMPS":dynamicdata)
                    n235 = Merge Signals(w164, w163) -> (→"LAB05 VOLTS":dynamicdata)
                    n236 = Merge Signals(w162, w160, w161, w159) -> (→"LAB05 TEMP":dynamicdata)
                    n237 = global write "Global display 3.vi" "graph flag"(FALSE) -> ()
                  }
                }
              }
            }
          }
          frame #2 {
            n238 = stacked-sequence {
              tunnel: 25 -> [w178 w215 w252 w289 w326 w363 w400 w437 w474 w511]
              frame #0 {
                n239 = local read "RUN LAB01-1"() -> (w179:bool)
                n240 = local read "LF1-1"() -> (w181:bool)
                n241 = Not(x=w179) -> (.not. x?=w182:bool)
                n242 = And(x=w182, y=w181) -> (x .and. y?=w180:bool)
                n243 = case shown="True" w180 {
                  tunnel: w178 -> [_ w183]
                  frame False {
                  }
                  frame True {
                    n244 = stacked-sequence {
                      tunnel: w183 -> [w184 _]
                      frame #0 {
                        n245 = flat-sequence {
                          tunnel: [w186] -> w185
                          tunnel: w185 -> [w189]
                          tunnel: w184 -> [w188]
                          frame #0 {
                            n246 = local read "log1-1"() -> (w187:dbl)
                            n247 = Increment(x=w187) -> (x+1=w186:dbl)
                            n248 = local write "log1-1"(w186) -> ()
                          }
                          frame #1 {
                            n249 = Greater?(x=w189, y=w188) -> (0:w190:bool)
                            n250 = case shown="True" w190 {
                              frame False {
                              }
                              frame True {
                                n251 = local write "LOG LAB01-1"("") -> ()
                                n252 = local write "log1-1"(0) -> ()
                              }
                            }
                          }
                        }
                      }
                      frame #1 {
                        w201 = "LAB01-1"
                        w205 = "/"
                        n253 = local read "DISP LAB01-1"() -> (w212:T4)
                        n254 = local read "SET LAB01-1"() -> (w206:T5)
                        n255 = Get Date/Time In Seconds() -> (seconds since 1Jan1904=w208:timestamp)
                        n256 = local write "LF1-1"(FALSE) -> ()
                        n257 = Unbundle(w206) -> ("DESCRIPTION"=w198:string)  [unwired: 4 out]
                        n258 = Unbundle(w212) -> ("CYCLE"=w211:dbl, "MINS"=w210:dbl, "STATUS"=w195:string)
                        n259 = Get Date/Time String(seconds (now)=w208) -> (date string=w200:string, time string=w199:string)  [unwired: 2 in]
                        n260 = local read "LOG LAB01-1"() -> (w204:string)
                        n261 = Number To Fractional String(number=w210, precision (6)=2) -> (F-format string=w196:string)  [unwired: 2 in]
                        n262 = Number To Decimal String(number=w211) -> (decimal integer string=w197:string)  [unwired: 1 in]
                        n263 = Bundle(w201, "date string"=w200, "time string"=w199, "DESCRIPTION"=w198, w197, w196, "STATUS"=w195) -> (w194:T7)  [unwired: 1 in]
                        n264 = Concatenate Strings(w201, w205, w200, w205, w199, w205, w198, w205, w197, w205, w196, w205, w195, "\r\n") -> (w202:string)
                        n265 = Concatenate Strings(w204, w202) -> (w203:string)
                        n266 = local write "LOG LAB01-1"(w203) -> ()
                        n267 = call "sub vi - Log udate V1.vi"("data"=w194, "panel id"=w201) -> ("error out"=→"error out":errorcluster)  [unwired: 9 in]
                      }
                    }
                  }
                }
                n268 = case shown="True" w179 {
                  frame False {
                  }
                  frame True {
                    n269 = local write "LF1-1"(TRUE) -> ()
                  }
                }
              }
              frame #1 {
                n270 = local read "RUN LAB01-2"() -> (w216:bool)
                n271 = local read "LF1-2"() -> (w218:bool)
                n272 = Not(x=w216) -> (.not. x?=w219:bool)
                n273 = And(x=w219, y=w218) -> (x .and. y?=w217:bool)
                n274 = case shown="True" w217 {
                  tunnel: w215 -> [_ w220]
                  frame False {
                  }
                  frame True {
                    n275 = stacked-sequence {
                      tunnel: w220 -> [w221 _]
                      frame #0 {
                        n276 = flat-sequence {
                          tunnel: [w223] -> w222
                          tunnel: w222 -> [w226]
                          tunnel: w221 -> [w225]
                          frame #0 {
                            n277 = local read "log1-2"() -> (w224:dbl)
                            n278 = Increment(x=w224) -> (x+1=w223:dbl)
                            n279 = local write "log1-2"(w223) -> ()
                          }
                          frame #1 {
                            n280 = Greater?(x=w226, y=w225) -> (0:w227:bool)
                            n281 = case shown="True" w227 {
                              frame False {
                              }
                              frame True {
                                n282 = local write "LOG LAB01-2"("") -> ()
                                n283 = local write "log1-2"(0) -> ()
                              }
                            }
                          }
                        }
                      }
                      frame #1 {
                        w238 = "LAB01-2"
                        w242 = "/"
                        n284 = local read "DISP LAB01-2"() -> (w249:T4)
                        n285 = local read "SET LAB01-2"() -> (w243:T5)
                        n286 = Get Date/Time In Seconds() -> (seconds since 1Jan1904=w245:timestamp)
                        n287 = local write "LF1-2"(FALSE) -> ()
                        n288 = Unbundle(w243) -> ("DESCRIPTION"=w235:string)  [unwired: 4 out]
                        n289 = Unbundle(w249) -> ("CYCLE"=w248:dbl, "MINS"=w247:dbl, "STATUS"=w232:string)
                        n290 = Get Date/Time String(seconds (now)=w245) -> (date string=w237:string, time string=w236:string)  [unwired: 2 in]
                        n291 = local read "LOG LAB01-2"() -> (w241:string)
                        n292 = Number To Fractional String(number=w247, precision (6)=2) -> (F-format string=w233:string)  [unwired: 2 in]
                        n293 = Number To Decimal String(number=w248) -> (decimal integer string=w234:string)  [unwired: 1 in]
                        n294 = Bundle(w238, "date string"=w237, "time string"=w236, "DESCRIPTION"=w235, w234, w233, "STATUS"=w232) -> (w231:T7)  [unwired: 1 in]
                        n295 = Concatenate Strings(w238, w242, w237, w242, w236, w242, w235, w242, w234, w242, w233, w242, w232, "\r\n") -> (w239:string)
                        n296 = Concatenate Strings(w241, w239) -> (w240:string)
                        n297 = local write "LOG LAB01-2"(w240) -> ()
                        n298 = call "sub vi - Log udate V1.vi"("data"=w231, "panel id"=w238) -> ("error out"=w230:errorcluster)  [unwired: 9 in]
                        n299 = local write "error out"(w230) -> ()
                      }
                    }
                  }
                }
                n300 = case shown="True" w216 {
                  frame False {
                  }
                  frame True {
                    n301 = local write "LF1-2"(TRUE) -> ()
                  }
                }
              }
              frame #2 {
                n302 = local read "RUN LAB02-1"() -> (w253:bool)
                n303 = local read "LF2-1"() -> (w255:bool)
                n304 = Not(x=w253) -> (.not. x?=w256:bool)
                n305 = And(x=w256, y=w255) -> (x .and. y?=w254:bool)
                n306 = case shown="True" w254 {
                  tunnel: w252 -> [_ w257]
                  frame False {
                  }
                  frame True {
                    n307 = stacked-sequence {
                      tunnel: w257 -> [w258 _]
                      frame #0 {
                        n308 = flat-sequence {
                          tunnel: [w260] -> w259
                          tunnel: w259 -> [w263]
                          tunnel: w258 -> [w262]
                          frame #0 {
                            n309 = local read "log2-1"() -> (w261:dbl)
                            n310 = Increment(x=w261) -> (x+1=w260:dbl)
                            n311 = local write "log2-1"(w260) -> ()
                          }
                          frame #1 {
                            n312 = Greater?(x=w263, y=w262) -> (0:w264:bool)
                            n313 = case shown="True" w264 {
                              frame False {
                              }
                              frame True {
                                n314 = local write "LOG LAB02-1"("") -> ()
                                n315 = local write "log2-1"(0) -> ()
                              }
                            }
                          }
                        }
                      }
                      frame #1 {
                        w275 = "LAB02-1"
                        w279 = "/"
                        n316 = local read "DISP LAB02-1"() -> (w286:T4)
                        n317 = local read "SET LAB02-1"() -> (w280:T5)
                        n318 = Get Date/Time In Seconds() -> (seconds since 1Jan1904=w282:timestamp)
                        n319 = local write "LF2-1"(FALSE) -> ()
                        n320 = Unbundle(w280) -> ("DESCRIPTION"=w272:string)  [unwired: 4 out]
                        n321 = Unbundle(w286) -> ("CYCLE"=w285:dbl, "MINS"=w284:dbl, "STATUS"=w269:string)
                        n322 = Get Date/Time String(seconds (now)=w282) -> (date string=w274:string, time string=w273:string)  [unwired: 2 in]
                        n323 = local read "LOG LAB02-1"() -> (w278:string)
                        n324 = Number To Fractional String(number=w284, precision (6)=2) -> (F-format string=w270:string)  [unwired: 2 in]
                        n325 = Number To Decimal String(number=w285) -> (decimal integer string=w271:string)  [unwired: 1 in]
                        n326 = Bundle(w275, "date string"=w274, "time string"=w273, "DESCRIPTION"=w272, w271, w270, "STATUS"=w269) -> (w268:T7)  [unwired: 1 in]
                        n327 = Concatenate Strings(w275, w279, w274, w279, w273, w279, w272, w279, w271, w279, w270, w279, w269, "\r\n") -> (w276:string)
                        n328 = Concatenate Strings(w278, w276) -> (w277:string)
                        n329 = local write "LOG LAB02-1"(w277) -> ()
                        n330 = call "sub vi - Log udate V1.vi"("data"=w268, "panel id"=w275) -> ("error out"=w267:errorcluster)  [unwired: 9 in]
                        n331 = local write "error out"(w267) -> ()
                      }
                    }
                  }
                }
                n332 = case shown="True" w253 {
                  frame False {
                  }
                  frame True {
                    n333 = local write "LF2-1"(TRUE) -> ()
                  }
                }
              }
              frame #3 {
                n334 = local read "RUN LAB02-2"() -> (w290:bool)
                n335 = local read "LF2-2"() -> (w292:bool)
                n336 = Not(x=w290) -> (.not. x?=w293:bool)
                n337 = And(x=w293, y=w292) -> (x .and. y?=w291:bool)
                n338 = case shown="True" w291 {
                  tunnel: w289 -> [_ w294]
                  frame False {
                  }
                  frame True {
                    n339 = stacked-sequence {
                      tunnel: w294 -> [w295 _]
                      frame #0 {
                        n340 = flat-sequence {
                          tunnel: [w297] -> w296
                          tunnel: w296 -> [w300]
                          tunnel: w295 -> [w299]
                          frame #0 {
                            n341 = local read "log2-2"() -> (w298:dbl)
                            n342 = Increment(x=w298) -> (x+1=w297:dbl)
                            n343 = local write "log2-2"(w297) -> ()
                          }
                          frame #1 {
                            n344 = Greater?(x=w300, y=w299) -> (0:w301:bool)
                            n345 = case shown="True" w301 {
                              frame False {
                              }
                              frame True {
                                n346 = local write "LOG LAB02-2"("") -> ()
                                n347 = local write "log2-2"(0) -> ()
                              }
                            }
                          }
                        }
                      }
                      frame #1 {
                        w312 = "LAB02-2"
                        w316 = "/"
                        n348 = local read "DISP LAB02-2"() -> (w323:T4)
                        n349 = local read "SET LAB02-2"() -> (w317:T5)
                        n350 = Get Date/Time In Seconds() -> (seconds since 1Jan1904=w319:timestamp)
                        n351 = local write "LF2-2"(FALSE) -> ()
                        n352 = Unbundle(w317) -> ("DESCRIPTION"=w309:string)  [unwired: 4 out]
                        n353 = Unbundle(w323) -> ("CYCLE"=w322:dbl, "MINS"=w321:dbl, "STATUS"=w306:string)
                        n354 = Get Date/Time String(seconds (now)=w319) -> (date string=w311:string, time string=w310:string)  [unwired: 2 in]
                        n355 = local read "LOG LAB02-2"() -> (w315:string)
                        n356 = Number To Fractional String(number=w321, precision (6)=2) -> (F-format string=w307:string)  [unwired: 2 in]
                        n357 = Number To Decimal String(number=w322) -> (decimal integer string=w308:string)  [unwired: 1 in]
                        n358 = Bundle(w312, "date string"=w311, "time string"=w310, "DESCRIPTION"=w309, w308, w307, "STATUS"=w306) -> (w305:T7)  [unwired: 1 in]
                        n359 = Concatenate Strings(w312, w316, w311, w316, w310, w316, w309, w316, w308, w316, w307, w316, w306, "\r\n") -> (w313:string)
                        n360 = Concatenate Strings(w315, w313) -> (w314:string)
                        n361 = local write "LOG LAB02-2"(w314) -> ()
                        n362 = call "sub vi - Log udate V1.vi"("data"=w305, "panel id"=w312) -> ("error out"=w304:errorcluster)  [unwired: 9 in]
                        n363 = local write "error out"(w304) -> ()
                      }
                    }
                  }
                }
                n364 = case shown="True" w290 {
                  frame False {
                  }
                  frame True {
                    n365 = local write "LF2-2"(TRUE) -> ()
                  }
                }
              }
              frame #4 {
                n366 = local read "RUN LAB03-1"() -> (w327:bool)
                n367 = local read "LF3-1"() -> (w329:bool)
                n368 = Not(x=w327) -> (.not. x?=w330:bool)
                n369 = And(x=w330, y=w329) -> (x .and. y?=w328:bool)
                n370 = case shown="True" w328 {
                  tunnel: w326 -> [_ w331]
                  frame False {
                  }
                  frame True {
                    n371 = stacked-sequence {
                      tunnel: w331 -> [w332 _]
                      frame #0 {
                        n372 = flat-sequence {
                          tunnel: [w334] -> w333
                          tunnel: w333 -> [w337]
                          tunnel: w332 -> [w336]
                          frame #0 {
                            n373 = local read "log3-1"() -> (w335:dbl)
                            n374 = Increment(x=w335) -> (x+1=w334:dbl)
                            n375 = local write "log3-1"(w334) -> ()
                          }
                          frame #1 {
                            n376 = Greater?(x=w337, y=w336) -> (0:w338:bool)
                            n377 = case shown="True" w338 {
                              frame False {
                              }
                              frame True {
                                n378 = local write "LOG LAB03-1"("") -> ()
                                n379 = local write "log3-1"(0) -> ()
                              }
                            }
                          }
                        }
                      }
                      frame #1 {
                        w349 = "LAB03-1"
                        w353 = "/"
                        n380 = local read "DISP LAB03-1"() -> (w360:T4)
                        n381 = local read "SET LAB03-1"() -> (w354:T5)
                        n382 = Get Date/Time In Seconds() -> (seconds since 1Jan1904=w356:timestamp)
                        n383 = local write "LF3-1"(FALSE) -> ()
                        n384 = Unbundle(w354) -> ("DESCRIPTION"=w346:string)  [unwired: 4 out]
                        n385 = Unbundle(w360) -> ("CYCLE"=w359:dbl, "MINS"=w358:dbl, "STATUS"=w343:string)
                        n386 = Get Date/Time String(seconds (now)=w356) -> (date string=w348:string, time string=w347:string)  [unwired: 2 in]
                        n387 = local read "LOG LAB03-1"() -> (w352:string)
                        n388 = Number To Fractional String(number=w358, precision (6)=2) -> (F-format string=w344:string)  [unwired: 2 in]
                        n389 = Number To Decimal String(number=w359) -> (decimal integer string=w345:string)  [unwired: 1 in]
                        n390 = Bundle(w349, "date string"=w348, "time string"=w347, "DESCRIPTION"=w346, w345, w344, "STATUS"=w343) -> (w342:T7)  [unwired: 1 in]
                        n391 = Concatenate Strings(w349, w353, w348, w353, w347, w353, w346, w353, w345, w353, w344, w353, w343, "\r\n") -> (w350:string)
                        n392 = Concatenate Strings(w352, w350) -> (w351:string)
                        n393 = local write "LOG LAB03-1"(w351) -> ()
                        n394 = call "sub vi - Log udate V1.vi"("data"=w342, "panel id"=w349) -> ("error out"=w341:errorcluster)  [unwired: 9 in]
                        n395 = local write "error out"(w341) -> ()
                      }
                    }
                  }
                }
                n396 = case shown="True" w327 {
                  frame False {
                  }
                  frame True {
                    n397 = local write "LF3-1"(TRUE) -> ()
                  }
                }
              }
              frame #5 {
                n398 = local read "RUN LAB03-2"() -> (w364:bool)
                n399 = local read "LF3-2"() -> (w366:bool)
                n400 = Not(x=w364) -> (.not. x?=w367:bool)
                n401 = And(x=w367, y=w366) -> (x .and. y?=w365:bool)
                n402 = case shown="True" w365 {
                  tunnel: w363 -> [_ w368]
                  frame False {
                  }
                  frame True {
                    n403 = stacked-sequence {
                      tunnel: w368 -> [w369 _]
                      frame #0 {
                        n404 = flat-sequence {
                          tunnel: [w371] -> w370
                          tunnel: w370 -> [w374]
                          tunnel: w369 -> [w373]
                          frame #0 {
                            n405 = local read "log3-2"() -> (w372:dbl)
                            n406 = Increment(x=w372) -> (x+1=w371:dbl)
                            n407 = local write "log3-2"(w371) -> ()
                          }
                          frame #1 {
                            n408 = Greater?(x=w374, y=w373) -> (0:w375:bool)
                            n409 = case shown="True" w375 {
                              frame False {
                              }
                              frame True {
                                n410 = local write "LOG LAB03-2"("") -> ()
                                n411 = local write "log3-2"(0) -> ()
                              }
                            }
                          }
                        }
                      }
                      frame #1 {
                        w386 = "LAB03-2"
                        w390 = "/"
                        n412 = local read "DISP LAB03-2"() -> (w397:T4)
                        n413 = local read "SET LAB03-2"() -> (w391:T5)
                        n414 = Get Date/Time In Seconds() -> (seconds since 1Jan1904=w393:timestamp)
                        n415 = local write "LF3-2"(FALSE) -> ()
                        n416 = Unbundle(w391) -> ("DESCRIPTION"=w383:string)  [unwired: 4 out]
                        n417 = Unbundle(w397) -> ("CYCLE"=w396:dbl, "MINS"=w395:dbl, "STATUS"=w380:string)
                        n418 = Get Date/Time String(seconds (now)=w393) -> (date string=w385:string, time string=w384:string)  [unwired: 2 in]
                        n419 = local read "LOG LAB03-2"() -> (w389:string)
                        n420 = Number To Fractional String(number=w395, precision (6)=2) -> (F-format string=w381:string)  [unwired: 2 in]
                        n421 = Number To Decimal String(number=w396) -> (decimal integer string=w382:string)  [unwired: 1 in]
                        n422 = Bundle(w386, "date string"=w385, "time string"=w384, "DESCRIPTION"=w383, w382, w381, "STATUS"=w380) -> (w379:T7)  [unwired: 1 in]
                        n423 = Concatenate Strings(w386, w390, w385, w390, w384, w390, w383, w390, w382, w390, w381, w390, w380, "\r\n") -> (w387:string)
                        n424 = Concatenate Strings(w389, w387) -> (w388:string)
                        n425 = local write "LOG LAB03-2"(w388) -> ()
                        n426 = call "sub vi - Log udate V1.vi"("data"=w379, "panel id"=w386) -> ("error out"=w378:errorcluster)  [unwired: 9 in]
                        n427 = local write "error out"(w378) -> ()
                      }
                    }
                  }
                }
                n428 = case shown="True" w364 {
                  frame False {
                  }
                  frame True {
                    n429 = local write "LF3-2"(TRUE) -> ()
                  }
                }
              }
              frame #6 {
                n430 = local read "RUN LAB04-1"() -> (w401:bool)
                n431 = local read "LF4-1"() -> (w403:bool)
                n432 = Not(x=w401) -> (.not. x?=w404:bool)
                n433 = And(x=w404, y=w403) -> (x .and. y?=w402:bool)
                n434 = case shown="True" w402 {
                  tunnel: w400 -> [_ w405]
                  frame False {
                  }
                  frame True {
                    n435 = stacked-sequence {
                      tunnel: w405 -> [w406 _]
                      frame #0 {
                        n436 = flat-sequence {
                          tunnel: [w408] -> w407
                          tunnel: w407 -> [w411]
                          tunnel: w406 -> [w410]
                          frame #0 {
                            n437 = local read "log4-1"() -> (w409:dbl)
                            n438 = Increment(x=w409) -> (x+1=w408:dbl)
                            n439 = local write "log4-1"(w408) -> ()
                          }
                          frame #1 {
                            n440 = Greater?(x=w411, y=w410) -> (0:w412:bool)
                            n441 = case shown="True" w412 {
                              frame False {
                              }
                              frame True {
                                n442 = local write "LOG LAB04-1"("") -> ()
                                n443 = local write "log4-1"(0) -> ()
                              }
                            }
                          }
                        }
                      }
                      frame #1 {
                        w423 = "LAB04-1"
                        w427 = "/"
                        n444 = local read "DISP LAB04-1"() -> (w434:T4)
                        n445 = local read "SET LAB04-1"() -> (w428:T5)
                        n446 = Get Date/Time In Seconds() -> (seconds since 1Jan1904=w430:timestamp)
                        n447 = local write "LF4-1"(FALSE) -> ()
                        n448 = Unbundle(w428) -> ("DESCRIPTION"=w420:string)  [unwired: 4 out]
                        n449 = Unbundle(w434) -> ("CYCLE"=w433:dbl, "MINS"=w432:dbl, "STATUS"=w417:string)
                        n450 = Get Date/Time String(seconds (now)=w430) -> (date string=w422:string, time string=w421:string)  [unwired: 2 in]
                        n451 = local read "LOG LAB04-1"() -> (w426:string)
                        n452 = Number To Fractional String(number=w432, precision (6)=2) -> (F-format string=w418:string)  [unwired: 2 in]
                        n453 = Number To Decimal String(number=w433) -> (decimal integer string=w419:string)  [unwired: 1 in]
                        n454 = Bundle(w423, "date string"=w422, "time string"=w421, "DESCRIPTION"=w420, w419, w418, "STATUS"=w417) -> (w416:T7)  [unwired: 1 in]
                        n455 = Concatenate Strings(w423, w427, w422, w427, w421, w427, w420, w427, w419, w427, w418, w427, w417, "\r\n") -> (w424:string)
                        n456 = Concatenate Strings(w426, w424) -> (w425:string)
                        n457 = local write "LOG LAB04-1"(w425) -> ()
                        n458 = call "sub vi - Log udate V1.vi"("data"=w416, "panel id"=w423) -> ("error out"=w415:errorcluster)  [unwired: 9 in]
                        n459 = local write "error out"(w415) -> ()
                      }
                    }
                  }
                }
                n460 = case shown="True" w401 {
                  frame False {
                  }
                  frame True {
                    n461 = local write "LF4-1"(TRUE) -> ()
                  }
                }
              }
              frame #7 {
                n462 = local read "RUN LAB04-2"() -> (w438:bool)
                n463 = local read "LF4-2"() -> (w440:bool)
                n464 = Not(x=w438) -> (.not. x?=w441:bool)
                n465 = And(x=w441, y=w440) -> (x .and. y?=w439:bool)
                n466 = case shown="True" w439 {
                  tunnel: w437 -> [_ w442]
                  frame False {
                  }
                  frame True {
                    n467 = stacked-sequence {
                      tunnel: w442 -> [w443 _]
                      frame #0 {
                        n468 = flat-sequence {
                          tunnel: [w445] -> w444
                          tunnel: w444 -> [w448]
                          tunnel: w443 -> [w447]
                          frame #0 {
                            n469 = local read "log4-2"() -> (w446:dbl)
                            n470 = Increment(x=w446) -> (x+1=w445:dbl)
                            n471 = local write "log4-2"(w445) -> ()
                          }
                          frame #1 {
                            n472 = Greater?(x=w448, y=w447) -> (0:w449:bool)
                            n473 = case shown="True" w449 {
                              frame False {
                              }
                              frame True {
                                n474 = local write "LOG LAB04-2"("") -> ()
                                n475 = local write "log4-2"(0) -> ()
                              }
                            }
                          }
                        }
                      }
                      frame #1 {
                        w460 = "LAB04-2"
                        w464 = "/"
                        n476 = local read "DISP LAB04-2"() -> (w471:T4)
                        n477 = local read "SET LAB04-2"() -> (w465:T5)
                        n478 = Get Date/Time In Seconds() -> (seconds since 1Jan1904=w467:timestamp)
                        n479 = local write "LF4-2"(FALSE) -> ()
                        n480 = Unbundle(w465) -> ("DESCRIPTION"=w457:string)  [unwired: 4 out]
                        n481 = Unbundle(w471) -> ("CYCLE"=w470:dbl, "MINS"=w469:dbl, "STATUS"=w454:string)
                        n482 = Get Date/Time String(seconds (now)=w467) -> (date string=w459:string, time string=w458:string)  [unwired: 2 in]
                        n483 = local read "LOG LAB04-2"() -> (w463:string)
                        n484 = Number To Fractional String(number=w469, precision (6)=2) -> (F-format string=w455:string)  [unwired: 2 in]
                        n485 = Number To Decimal String(number=w470) -> (decimal integer string=w456:string)  [unwired: 1 in]
                        n486 = Bundle(w460, "date string"=w459, "time string"=w458, "DESCRIPTION"=w457, w456, w455, "STATUS"=w454) -> (w453:T7)  [unwired: 1 in]
                        n487 = Concatenate Strings(w460, w464, w459, w464, w458, w464, w457, w464, w456, w464, w455, w464, w454, "\r\n") -> (w461:string)
                        n488 = Concatenate Strings(w463, w461) -> (w462:string)
                        n489 = local write "LOG LAB04-2"(w462) -> ()
                        n490 = call "sub vi - Log udate V1.vi"("data"=w453, "panel id"=w460) -> ("error out"=w452:errorcluster)  [unwired: 9 in]
                        n491 = local write "error out"(w452) -> ()
                      }
                    }
                  }
                }
                n492 = case shown="True" w438 {
                  frame False {
                  }
                  frame True {
                    n493 = local write "LF4-2"(TRUE) -> ()
                  }
                }
              }
              frame #8 {
                n494 = local read "RUN LAB05-1"() -> (w475:bool)
                n495 = local read "LF5-1"() -> (w477:bool)
                n496 = Not(x=w475) -> (.not. x?=w478:bool)
                n497 = And(x=w478, y=w477) -> (x .and. y?=w476:bool)
                n498 = case shown="True" w476 {
                  tunnel: w474 -> [_ w479]
                  frame False {
                  }
                  frame True {
                    n499 = stacked-sequence {
                      tunnel: w479 -> [w480 _]
                      frame #0 {
                        n500 = flat-sequence {
                          tunnel: [w482] -> w481
                          tunnel: w481 -> [w485]
                          tunnel: w480 -> [w484]
                          frame #0 {
                            n501 = local read "log5-1"() -> (w483:dbl)
                            n502 = Increment(x=w483) -> (x+1=w482:dbl)
                            n503 = local write "log5-1"(w482) -> ()
                          }
                          frame #1 {
                            n504 = Greater?(x=w485, y=w484) -> (0:w486:bool)
                            n505 = case shown="True" w486 {
                              frame False {
                              }
                              frame True {
                                n506 = local write "LOG LAB05-1"("") -> ()
                                n507 = local write "log5-1"(0) -> ()
                              }
                            }
                          }
                        }
                      }
                      frame #1 {
                        w497 = "LAB05-1"
                        w501 = "/"
                        n508 = local read "DISP LAB05-1"() -> (w508:T4)
                        n509 = local read "SET LAB05-1"() -> (w502:T5)
                        n510 = Get Date/Time In Seconds() -> (seconds since 1Jan1904=w504:timestamp)
                        n511 = local write "LF5-1"(FALSE) -> ()
                        n512 = Unbundle(w502) -> ("DESCRIPTION"=w494:string)  [unwired: 4 out]
                        n513 = Unbundle(w508) -> ("CYCLE"=w507:dbl, "MINS"=w506:dbl, "STATUS"=w491:string)
                        n514 = Get Date/Time String(seconds (now)=w504) -> (date string=w496:string, time string=w495:string)  [unwired: 2 in]
                        n515 = local read "LOG LAB05-1"() -> (w500:string)
                        n516 = Number To Fractional String(number=w506, precision (6)=2) -> (F-format string=w492:string)  [unwired: 2 in]
                        n517 = Number To Decimal String(number=w507) -> (decimal integer string=w493:string)  [unwired: 1 in]
                        n518 = Bundle(w497, "date string"=w496, "time string"=w495, "DESCRIPTION"=w494, w493, w492, "STATUS"=w491) -> (w490:T7)  [unwired: 1 in]
                        n519 = Concatenate Strings(w497, w501, w496, w501, w495, w501, w494, w501, w493, w501, w492, w501, w491, "\r\n") -> (w498:string)
                        n520 = Concatenate Strings(w500, w498) -> (w499:string)
                        n521 = local write "LOG LAB05-1"(w499) -> ()
                        n522 = call "sub vi - Log udate V1.vi"("data"=w490, "panel id"=w497) -> ("error out"=w489:errorcluster)  [unwired: 9 in]
                        n523 = local write "error out"(w489) -> ()
                      }
                    }
                  }
                }
                n524 = case shown="True" w475 {
                  frame False {
                  }
                  frame True {
                    n525 = local write "LF5-1"(TRUE) -> ()
                  }
                }
              }
              frame #9 {
                n526 = local read "RUN LAB05-2"() -> (w512:bool)
                n527 = local read "LF5-2"() -> (w514:bool)
                n528 = Not(x=w512) -> (.not. x?=w515:bool)
                n529 = And(x=w515, y=w514) -> (x .and. y?=w513:bool)
                n530 = case shown="True" w513 {
                  tunnel: w511 -> [_ w516]
                  frame False {
                  }
                  frame True {
                    n531 = stacked-sequence {
                      tunnel: w516 -> [w517 _]
                      frame #0 {
                        n532 = flat-sequence {
                          tunnel: [w519] -> w518
                          tunnel: w518 -> [w522]
                          tunnel: w517 -> [w521]
                          frame #0 {
                            n533 = local read "log5-2"() -> (w520:dbl)
                            n534 = Increment(x=w520) -> (x+1=w519:dbl)
                            n535 = local write "log5-2"(w519) -> ()
                          }
                          frame #1 {
                            n536 = Greater?(x=w522, y=w521) -> (0:w523:bool)
                            n537 = case shown="True" w523 {
                              frame False {
                              }
                              frame True {
                                n538 = local write "LOG LAB05-2"("") -> ()
                                n539 = local write "log5-2"(0) -> ()
                              }
                            }
                          }
                        }
                      }
                      frame #1 {
                        w534 = "LAB05-2"
                        w538 = "/"
                        n540 = local read "DISP LAB05-2"() -> (w545:T4)
                        n541 = local read "SET LAB05-2"() -> (w539:T5)
                        n542 = Get Date/Time In Seconds() -> (seconds since 1Jan1904=w541:timestamp)
                        n543 = local write "LF5-2"(FALSE) -> ()
                        n544 = Unbundle(w539) -> ("DESCRIPTION"=w531:string)  [unwired: 4 out]
                        n545 = Unbundle(w545) -> ("CYCLE"=w544:dbl, "MINS"=w543:dbl, "STATUS"=w528:string)
                        n546 = Get Date/Time String(seconds (now)=w541) -> (date string=w533:string, time string=w532:string)  [unwired: 2 in]
                        n547 = local read "LOG LAB05-2"() -> (w537:string)
                        n548 = Number To Fractional String(number=w543, precision (6)=2) -> (F-format string=w529:string)  [unwired: 2 in]
                        n549 = Number To Decimal String(number=w544) -> (decimal integer string=w530:string)  [unwired: 1 in]
                        n550 = Bundle(w534, "date string"=w533, "time string"=w532, "DESCRIPTION"=w531, w530, w529, "STATUS"=w528) -> (w527:T7)  [unwired: 1 in]
                        n551 = Concatenate Strings(w534, w538, w533, w538, w532, w538, w531, w538, w530, w538, w529, w538, w528, "\r\n") -> (w535:string)
                        n552 = Concatenate Strings(w537, w535) -> (w536:string)
                        n553 = local write "LOG LAB05-2"(w536) -> ()
                        n554 = call "sub vi - Log udate V1.vi"("data"=w527, "panel id"=w534) -> ("error out"=w526:errorcluster)  [unwired: 9 in]
                        n555 = local write "error out"(w526) -> ()
                      }
                    }
                  }
                }
                n556 = case shown="True" w512 {
                  frame False {
                  }
                  frame True {
                    n557 = local write "LF5-2"(TRUE) -> ()
                  }
                }
              }
            }
          }
          frame #3 {
            # "save current log files to network dir for viewing"
            # "save last months log files to networ dir for new month"
            # "send log data to main program"
            n558 = local read "LOG LAB05-2"() -> (w562:string)
            n559 = local read "LOG LAB02-1"() -> (w569:string)
            n560 = local read "LOG LAB03-2"() -> (w566:string)
            n561 = local read "LOG LAB04-1"() -> (w565:string)
            n562 = local read "LOG LAB05-1"() -> (w563:string)
            n563 = local read "LOG LAB02-2"() -> (w568:string)
            n564 = local read "LOG LAB04-2"() -> (w564:string)
            n565 = local read "LOG LAB03-1"() -> (w567:string)
            n566 = local read "LOG LAB01-2"() -> (w570:string)
            n567 = local read "LOG LAB01-1"() -> (w571:string)
            n568 = global write "Global display 3.vi" "log 5-2"(w562) -> ()
            n569 = global write "Global display 3.vi" "log 4-2"(w564) -> ()
            n570 = global write "Global display 3.vi" "log 1-1"(w571) -> ()
            n571 = global write "Global display 3.vi" "log 5-1"(w563) -> ()
            n572 = global write "Global display 3.vi" "log 1-2"(w570) -> ()
            n573 = global write "Global display 3.vi" "log 4-1"(w565) -> ()
            n574 = global write "Global display 3.vi" "log 2-2"(w568) -> ()
            n575 = global write "Global display 3.vi" "log 2-1"(w569) -> ()
            n576 = global write "Global display 3.vi" "log 3-1"(w567) -> ()
            n577 = global write "Global display 3.vi" "log 3-2"(w566) -> ()
            n578 = property on="Tab Control 2" class="TabCtl (strict)"() -> ("Pages"=w551:refnum<vi>[])  [unwired: 2 in, 2 out]
            n579 = global read "Global display 3.vi" "admin"() -> (w548:bool)
            n580 = Index Array(array=w551, index=8) -> (element=w549:refnum<vi>)
            n581 = property class="Page"(reference=w549, "PageVis"=w548) -> ()  [unwired: 1 in, 2 out]
            n582 = Get Date/Time In Seconds() -> (seconds since 1Jan1904=w559:timestamp)
            n583 = case shown="True" "Save Log Files\nTo Disk For\nViewing" {
              frame False {
              }
              frame True {
                n584 = stacked-sequence {
                  seq-local: [w576 _] -> [_ w579]
                  frame #0 {
                    n585 = call "sub vi - save log files V1.vi"() -> ("network dir"=w576:string)  [unwired: 10 in]
                  }
                  frame #1 {
                    n586 = local write "Save Log Files\nTo Disk For\nViewing"(FALSE) -> ()
                    n587 = Concatenate Strings("Saved:", w579) -> (w578:string)
                    n588 = One Button Dialog(message=w578) -> ()  [unwired: 1 in, 1 out]
                  }
                }
              }
            }
            n589 = Format Date/Time String(time format string (%c)="\\LabPanel%Y\\%b", seconds (now)=w559) -> (date/time string=w552:string)  [unwired: 1 in]
            n590 = local read "log file dir"() -> (w556:string)
            n591 = Equal?(x=w556, y="") -> (x = y?=w557:bool)
            n592 = Select(t=w552, s=w557, f=w556) -> (s? t:f=→"log file dir":string)
            n593 = local read "log file dir"() -> (w553:string)
            n594 = Not Equal?(x=w552, y=w553) -> (x != y?=w554:bool)
            n595 = case shown="True" w554 {
              tunnel: w553 -> [_ w573]
              tunnel: w552 -> [_ w572]
              frame False {
              }
              frame True {
                n596 = stacked-sequence {
                  tunnel: w573 -> [w574 _]
                  tunnel: w572 -> [_ w575]
                  frame #0 {
                    n597 = call "sub vi - save log dir V1.vi"("Dir Input"=w574) -> ()  [unwired: 11 in]
                  }
                  frame #1 {
                    n598 = local write "log file dir"(w575) -> ()
                  }
                }
              }
            }
          }
        }
        n599 = global read "Global display 1.vi" "stop disp"() -> (w2:bool)
        n600 = Or(x="Stop Button", y=w2) -> (x .or. y?=w4:bool)
      }
    }
  }
